vi "Write ip.vi"(8 "error in (no error)":errorcluster, 10 "ip":string="localhost", 11 "Server in":refnum<class "TCP-Server.lvclass">) -> (0 "error out":errorcluster, 3 "Server out":refnum<class "TCP-Server.lvclass">)   [LabVIEW 2018, in "TCP-Server.lvclass"]
uses:
  TCP-Server.lvclass
  TCP-Server.lvclass/TCP-Server.ctl
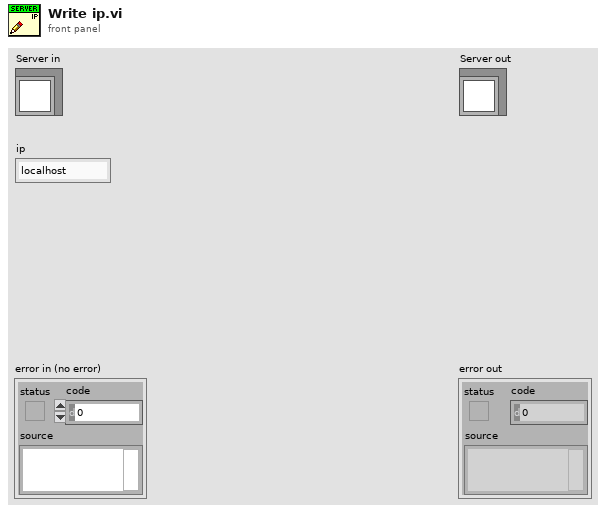
[diagram p1: front panel]
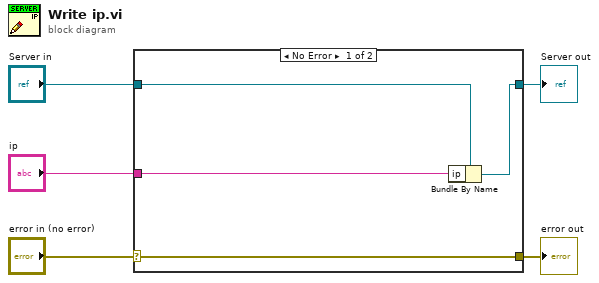
[diagram p0: block diagram]
diagram:
  n1 = case shown="No Error" "error in (no error)" {
    selector: "error in (no error)" -> [w9 w10]
    tunnel: [w9 w10] -> w4
    tunnel: [w7 w11] -> w2
    tunnel: "Server in" -> [w8 w11]
    tunnel: "ip" -> [w6 _]
    frame No Error {
      n2 = Bundle By Name(cluster=w8, "ip"=w6) -> (w7:refnum<class "TCP-Server.lvclass">)
    }
    frame Error {
    }
  }
  "error out" <- w4
  "Server out" <- w2
